vi "CD Read Engine_Parse Message_Update Channels.vi"(8 "error in (no error)":errorcluster, 9 "NORESP":bool, 10 "Frame Descriptor":T2 {"RT"."Status Channel Ref" format="%.0x"; "RT"."Words Block Data Refs"."Data Reference" format="%.0x"; "RT"."Timestamp Channel Data Reference" format="%.0x"; "BC"."Status Channel Refs" format="%.0x"; "BC"."Words Block Data Refs"."Data Reference" format="%.0x"; "BC"."Timestamp Channel Data Reference" format="%.0x"}, 11 "record in":T1 {"type" format="%04x"; "activity" format="%04x"; "error" format="%04x"; "cwd1" format="%04x"; "cwd2" format="%04x"; "swd1" format="%04x"; "swd2" format="%04x"; "data" format="%04x"}) -> (0 "error out":errorcluster, 3 "Timestamp (s)":dbl)   [LabVIEW 2017, in "Ballard MIL-1553 Engine.lvlib"]
uses:
  Ballard MIL-1553 Engine.lvlib
  Controls/RT Inline Frame Descriptor.ctl
  Controls/RT Inline Frame Descriptor_BC.ctl
  <vilib>/NI Veristand/Custom Device API/Data Reference.ctl
  <vilib>/NI Veristand/Custom Device API/Block Data Reference.ctl
  <vilib>/NI Veristand/Custom Device API/Custom Device Item Ref.ctl
  Controls/RT Inline Frame Descriptor_RT.ctl
  Shared/Controls and Global/RT CWD2.ctl
  Shared/Controls and Global/RT CWD1.ctl
  Shared/Controls and Global/RT messageType.ctl
  <instrlib>/BTICardLib/Public/Controls/1553 Record.ctl
  <vilib>/NI Veristand/Custom Device API/Global Data Refs.vi
  <vilib>/NI VeriStand/Custom Device API/Custom Device API.lvlib
  Shared/Ballard 1553 Shared.lvlib
  <vilib>/NI VeriStand/Custom Device Tools/Custom Device Utility Library/Custom Device Utility Library.lvlib
  <instrlib>/BTICardLib/BTICardLV.lvlib
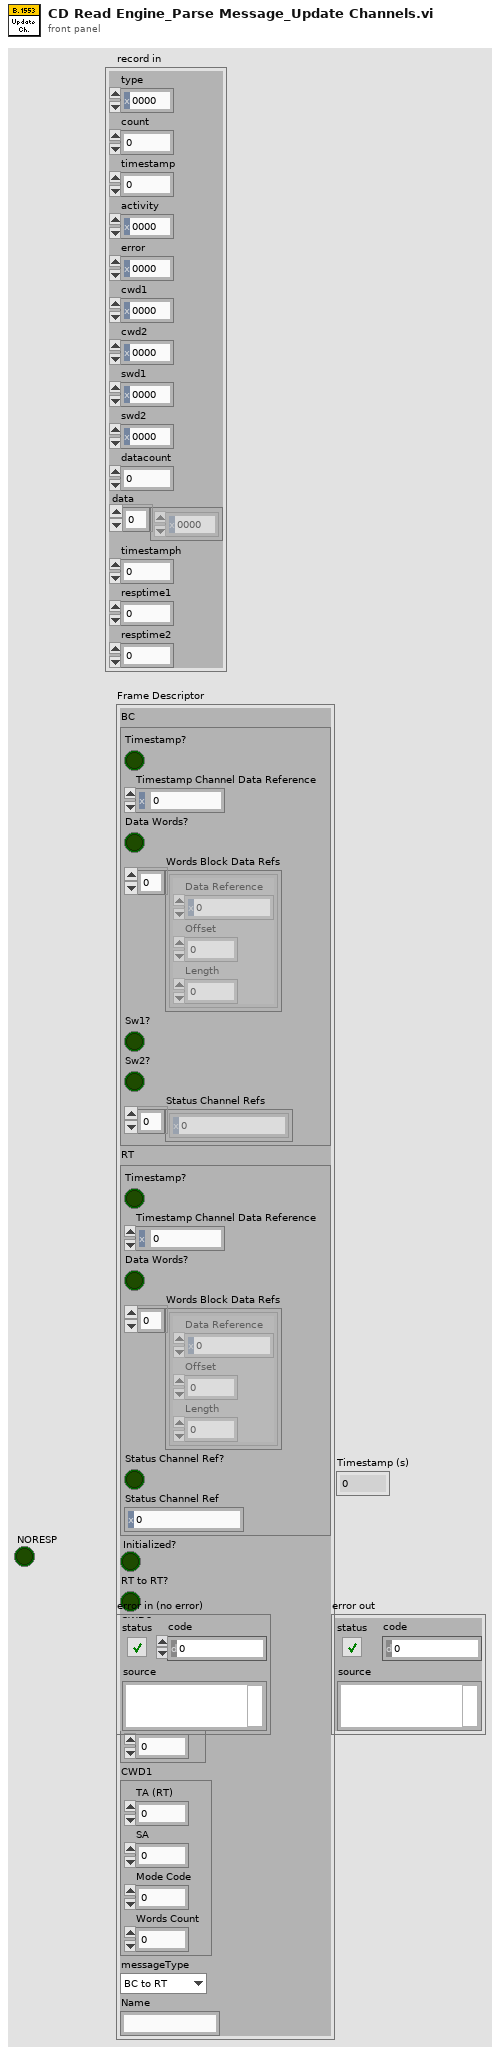
[diagram p1: front panel]
types:
  T1 = typedef "BTICardLV.lvlib/1553 Record.ctl" = cluster{"type":u16, "count":u16, "timestamp":u32, "activity":u16, "error":u16, "cwd1":u16, "cwd2":u16, "swd1":u16, "swd2":u16, "datacount":u16, "data":u16[], "timestamph":u32, "resptime1":u16, "resptime2":u16}
  T2 = typedef "Ballard MIL-1553 Engine.lvlib/RT Inline Frame Descriptor.ctl" = cluster{"BC":T3, "RT":T7, "Initialized?":bool, "RT to RT?":bool, "CWD2":T8, "CWD1":T9, "messageType":T10, "Name":string}
  T3 = typedef "Ballard MIL-1553 Engine.lvlib/RT Inline Frame Descriptor_BC.ctl" = cluster{"Timestamp?":bool, "Timestamp Channel Data Reference":T4, "Data Words?":bool, "Words Block Data Refs":T5[], "Sw1?":bool, "Sw2?":bool, "Status Channel Refs":T6[]}
  T4 = typedef "Custom Device API.lvlib/Data Reference.ctl" = i32
  T5 = typedef "Custom Device API.lvlib/Block Data Reference.ctl" = cluster{"Data Reference":T4, "Offset":u64, "Length":u64}
  T6 = typedef "Custom Device API.lvlib/Custom Device Item Ref.ctl" = u64
  T7 = typedef "Ballard MIL-1553 Engine.lvlib/RT Inline Frame Descriptor_RT.ctl" = cluster{"Timestamp?":bool, "Timestamp Channel Data Reference":T4, "Data Words?":bool, "Words Block Data Refs":T5[], "Status Channel Ref?":bool, "Status Channel Ref":T6}
  T8 = typedef "Ballard 1553 Shared.lvlib/RT CWD2.ctl" = cluster{"TA (RT)":i8, "SA":i8, "Words (WC)":i8}
  T9 = typedef "Ballard 1553 Shared.lvlib/RT CWD1.ctl" = cluster{"TA (RT)":i8, "SA":i8, "Mode Code":i8, "Words Count":i8}
  T10 = typedef "Ballard 1553 Shared.lvlib/RT messageType.ctl" = enum16{"BC to RT", "RT to BC", "RT to RT", "MC (Rx)", "MC (Tx)"}
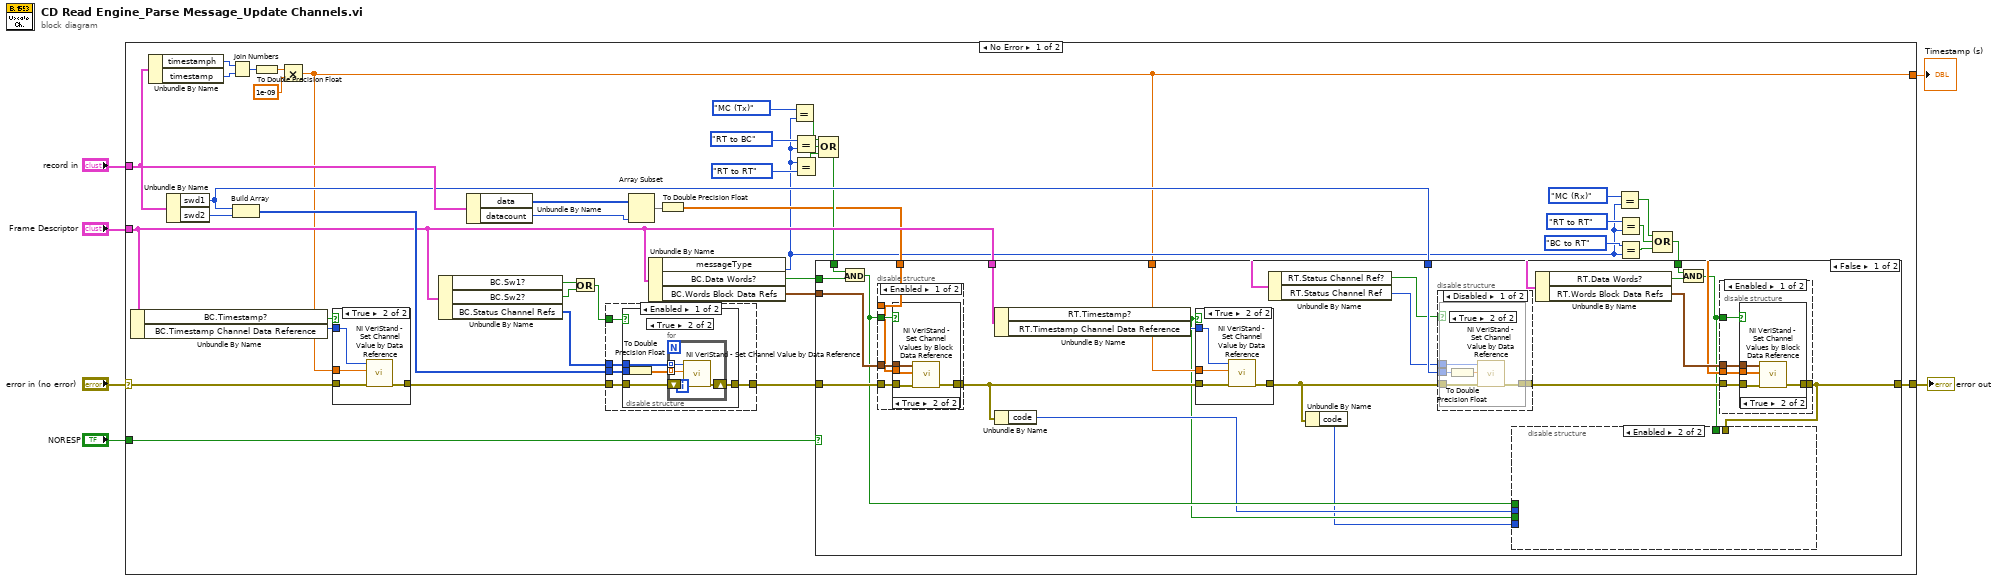
[diagram p0: block diagram]
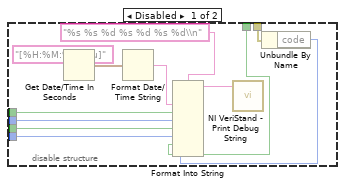
[diagram p2: hidden frame]
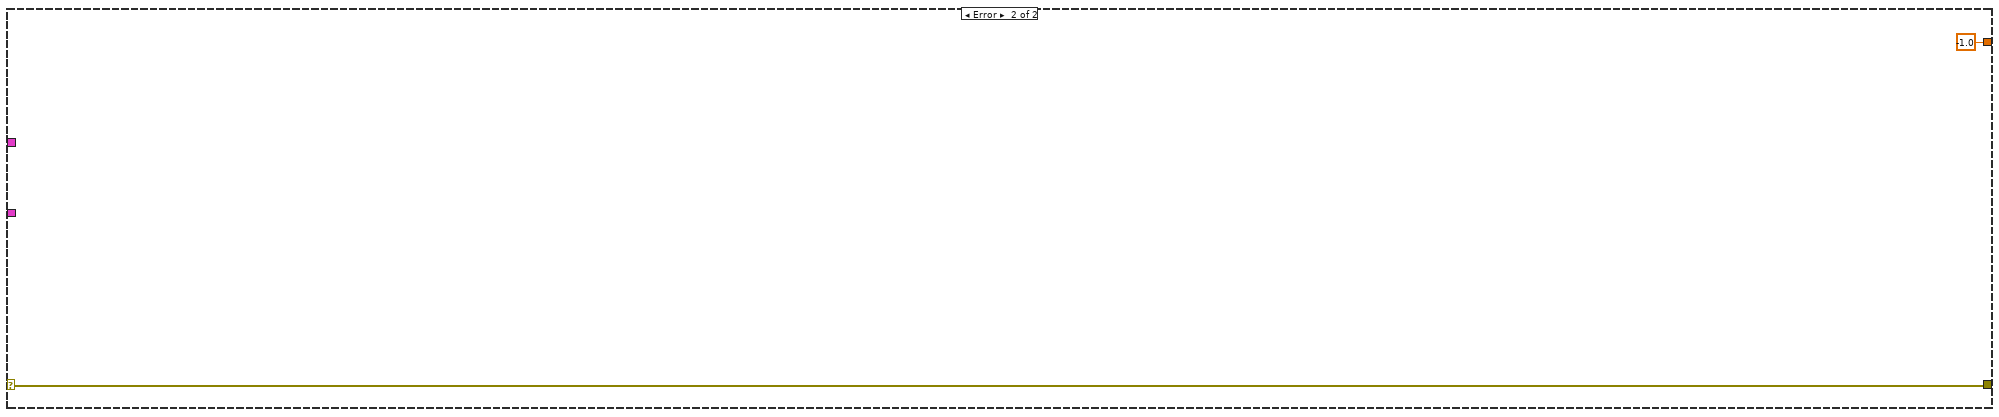
[diagram p14: hidden frame]
diagram:
  n1 = case shown="No Error" "error in (no error)" {
    selector: "error in (no error)" -> [w42 w146]
    tunnel: "Frame Descriptor" -> [w36 _]
    tunnel: [w37 w146] -> w5
    tunnel: "record in" -> [w38 _]
    tunnel: "NORESP" -> [w14 _]
    tunnel: [w7 -1.0] -> w1
    frame No Error {
      n2 = Unbundle By Name(w36) -> ("BC.Timestamp?"=w44:bool, "BC.Timestamp Channel Data Reference"=w43:T4)
      n3 = Unbundle By Name(w38) -> ("timestamph"=w45:u32, "timestamp"=w46:u32)
      n4 = Unbundle By Name(w38) -> ("swd1"=w35:u16, "swd2"=w40:u16)
      n5 = Join Numbers(hi=w45, lo=w46) -> ((hi.lo)=w47:u64)
      n6 = Build Array(w35, w40) -> (w39:u16[])
      n7 = To Double Precision Float(number=w47) -> (double precision float=w48:dbl)
      n8 = Multiply(x=w48, y=1e-09) -> (x*y=w7:dbl)
      n9 = case shown="True" w44 {
        tunnel: w43 -> [_ w144]
        tunnel: w7 -> [_ w143]
        tunnel: w42 -> [w140 w142]
        tunnel: [w140 w141] -> w41
        frame False {
        }
        frame True {
          n10 = call <vilib>:"NI VeriStand - Set Channel Value by Data Reference.vi"("error in (no error)"=w142, "Value"=w143, "Data Reference in"=w144) -> ("error out"=w141:errorcluster)  [unwired: 8 in]
        }
      }
      n11 = Unbundle By Name(w36) -> ("BC.Sw1?"=w33:bool, "BC.Sw2?"=w34:bool, "BC.Status Channel Refs"=w31:T6[])
      n12 = Unbundle By Name(w38) -> ("data"=w28:u16[], "datacount"=w15:u16)
      n13 = Or(x=w33, y=w34) -> (x .or. y?=w32:bool)
      n14 = disable-structure shown="Enabled" {
        disable-tunnel: w41 -> [w128 w139]
        disable-tunnel: w39 -> [w127 _]
        disable-tunnel: w32 -> [w126 _]
        disable-tunnel: w31 -> [w125 _]
        disable-tunnel: [w124 w139] -> w30
        frame Enabled {
          n15 = case shown="True" w126 {
            tunnel: w125 -> [_ w134]
            tunnel: w127 -> [_ w133]
            tunnel: w128 -> [w129 w132]
            tunnel: [w129 w131] -> w124
            frame False {
            }
            frame True {
              n16 = To Double Precision Float(number=w133) -> (double precision float=w130:dbl[])
              n17 = for {
                tunnel: w134 -> [w138] mode=indexing
                tunnel: w130 -> [w137] mode=indexing
                shift-right: [w135] -> w131
                shift-left: w132 -> [w136]
                n18 = call <vilib>:"NI VeriStand - Set Channel Value by Data Reference.vi"("error in (no error)"=w136, "Value"=w137, "Data Reference in"=w138) -> ("error out"=w135:errorcluster)  [unwired: 8 in]
              }
            }
          }
        }
        frame Disabled {
        }
      }
      n19 = Array Subset(array=w28, length=w15) -> (w27:u16[])  [unwired: 1 in]
      n20 = Unbundle By Name(w36) -> ("messageType"=w8:T10, "BC.Data Words?"=w19:bool, "BC.Words Block Data Refs"=w29:T5[])
      n21 = To Double Precision Float(number=w27) -> (double precision float=w16:dbl[])
      n22 = Equal?(x=RT_messageType."MC (Tx)", y=w8) -> (x = y?=w9:bool)
      n23 = Equal?(x=RT_messageType."RT to BC", y=w8) -> (x = y?=w21:bool)
      n24 = Equal?(x=w8, y=RT_messageType."RT to RT") -> (x = y?=w20:bool)
      n25 = Compound Arithmetic op=OR(w9, w21, w20) -> (w25:bool)
      n26 = Equal?(x=RT_messageType."MC (Rx)", y=w8) -> (x = y?=w11:bool)
      n27 = Equal?(x=RT_messageType."RT to RT", y=w8) -> (x = y?=w18:bool)
      n28 = Equal?(x=RT_messageType."BC to RT", y=w8) -> (x = y?=w17:bool)
      n29 = Compound Arithmetic op=OR(w11, w18, w17) -> (w23:bool)
      n30 = case shown="False" w14 {
        tunnel: w7 -> [w72 _]
        tunnel: [w50 w123] -> w37
        tunnel: w36 -> [w71 _]
        tunnel: w35 -> [w70 _]
        tunnel: w30 -> [w69 w123]
        tunnel: w29 -> [w68 _]
        tunnel: w25 -> [w62 _]
        tunnel: w23 -> [w61 _]
        tunnel: w19 -> [w60 _]
        tunnel: w16 -> [w58 _]
        frame False {
          n31 = And(x=w62, y=w60) -> (x .and. y?=w57:bool)
          n32 = disable-structure shown="Enabled" {
            disable-tunnel: w57 -> [w111 _]
            disable-tunnel: w69 -> [w110 w117]
            disable-tunnel: w68 -> [w109 _]
            disable-tunnel: [w108 w117] -> w56
            disable-tunnel: w58 -> [w107 _]
            frame Enabled {
              n33 = case shown="True" w111 {
                tunnel: w110 -> [w112 w116]
                tunnel: w109 -> [_ w115]
                tunnel: w107 -> [_ w114]
                tunnel: [w112 w113] -> w108
                frame False {
                }
                frame True {
                  n34 = call <vilib>:"NI VeriStand - Set Channel Values by Block Data Reference.vi"("error in (no error)"=w116, "Values Array in"=w114, "Block Data Ref"=w115) -> ("error out"=w113:errorcluster)  [unwired: 6 in, 2 out]
                }
              }
            }
            frame Disabled {
            }
          }
          n35 = Unbundle By Name(w71) -> ("RT.Timestamp?"=w53:bool, "RT.Timestamp Channel Data Reference"=w66:T4)
          n36 = Unbundle By Name(w56) -> ("code"=w54:i32)
          n37 = case shown="True" w53 {
            tunnel: w66 -> [_ w122]
            tunnel: w72 -> [_ w121]
            tunnel: w56 -> [w118 w120]
            tunnel: [w118 w119] -> w55
            frame False {
            }
            frame True {
              n38 = call <vilib>:"NI VeriStand - Set Channel Value by Data Reference.vi"("error in (no error)"=w120, "Value"=w121, "Data Reference in"=w122) -> ("error out"=w119:errorcluster)  [unwired: 8 in]
            }
          }
          n39 = Unbundle By Name(w71) -> ("RT.Status Channel Ref?"=w64:bool, "RT.Status Channel Ref"=w65:T6)
          n40 = Unbundle By Name(w55) -> ("code"=w52:i32)
          n41 = disable-structure shown="Disabled" {
            disable-tunnel: w70 -> [w99 _]
            disable-tunnel: w65 -> [w98 _]
            disable-tunnel: w64 -> [w97 _]
            disable-tunnel: w55 -> [w96 w106]
            disable-tunnel: [w95 w106] -> w63
            frame Disabled {
              n42 = case shown="True" w97 {
                tunnel: w98 -> [_ w103]
                tunnel: [w100 w104] -> w95
                tunnel: w96 -> [w100 w105]
                tunnel: w99 -> [_ w102]
                frame False {
                }
                frame True {
                  n43 = To Double Precision Float(number=w102) -> (double precision float=w101:dbl)
                  n44 = call <vilib>:"NI VeriStand - Set Channel Value by Data Reference.vi"("error in (no error)"=w105, "Value"=w101, "Data Reference in"=w103) -> ("error out"=w104:errorcluster)  [unwired: 8 in]
                }
              }
            }
            frame Enabled {
            }
          }
          n45 = Unbundle By Name(w71) -> ("RT.Data Words?"=w59:bool, "RT.Words Block Data Refs"=w67:T5[])
          n46 = And(x=w61, y=w59) -> (x .and. y?=w51:bool)
          n47 = disable-structure shown="Enabled" {
            disable-tunnel: [w88 w94] -> w50
            disable-tunnel: w67 -> [w87 _]
            disable-tunnel: w51 -> [w86 _]
            disable-tunnel: w58 -> [w85 _]
            disable-tunnel: w63 -> [w84 w94]
            frame Enabled {
              n48 = case shown="True" w86 {
                tunnel: w84 -> [w89 w93]
                tunnel: w87 -> [_ w92]
                tunnel: [w89 w91] -> w88
                tunnel: w85 -> [_ w90]
                frame False {
                }
                frame True {
                  n49 = call <vilib>:"NI VeriStand - Set Channel Values by Block Data Reference.vi"("error in (no error)"=w93, "Values Array in"=w90, "Block Data Ref"=w92) -> ("error out"=w91:errorcluster)  [unwired: 6 in, 2 out]
                }
              }
            }
            frame Disabled {
            }
          }
          n50 = disable-structure shown="Enabled" {
            disable-tunnel: w57 -> [w79 _]
            disable-tunnel: w54 -> [w78 _]
            disable-tunnel: w53 -> [w77 _]
            disable-tunnel: w52 -> [w76 _]
            disable-tunnel: w51 -> [w75 _]
            disable-tunnel: w50 -> [w73 _]
            frame Disabled {
              (unwired) "[%H:%M:%S%3u]" ("time format string (%c)")
              n51 = Get Date/Time In Seconds() -> (seconds since 1Jan1904=w82:timestamp)
              n52 = Format Date/Time String(seconds (now)=w82) -> (date/time string=w81:string)  [unwired: 2 in]
              n53 = Unbundle By Name(w73) -> ("code"=w74:i32)
              n54 = Format Into String(format string="%s %s %d %s %d %s %d\\n", w81, w79, w78, w77, w76, w75, w74) -> (resulting string=w83:string)  [unwired: 2 in, 1 out]
              n55 = call <vilib>:"NI VeriStand - Print Debug String.vi"("Message"=w83) -> ()  [unwired: 10 in, 1 out]
            }
            frame Enabled {
            }
          }
        }
        frame True {
          # "NO RESPONSE from RT."
        }
      }
    }
    frame Error {
    }
  }
  "error out" <- w5
  "Timestamp (s)" <- w1
